vi "WriteMultipleReg.vi"(5 "DAC电压值":dbl min=0.0 max=3.3 step=0.1) -> (2 "数组":u16[](array[numeric]))   [LabVIEW 2013]
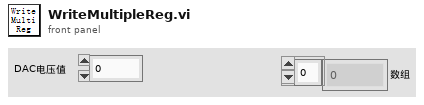
[diagram p1: front panel]
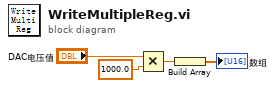
[diagram p0: block diagram]
diagram:
  n1 = Multiply(x="DAC电压值", y=1000.0) -> (x*y=w2:dbl)
  n2 = Build Array(w2) -> (→"数组":dbl[])
